vi "Disconnect.vi"(8 "error in (no error)":errorcluster, 11 "Ref":T1) -> (0 "error out":errorcluster)   [LabVIEW 2019, in "Ghost Bus Host Automation API.lvlib"]
uses:
  Ghost Bus Host Automation API.lvlib
  <vilib>/NI/STM/NI STM.lvlib
  <vilib>/NI/STM/TCP/Get Connection Reference (TCP).vi
  <vilib>/NI/STM/SubVIs/MetaDataElement.ctl
  <vilib>/NI/STM/TCP/TCP Connection Info.ctl
  Types/API Variables.ctl
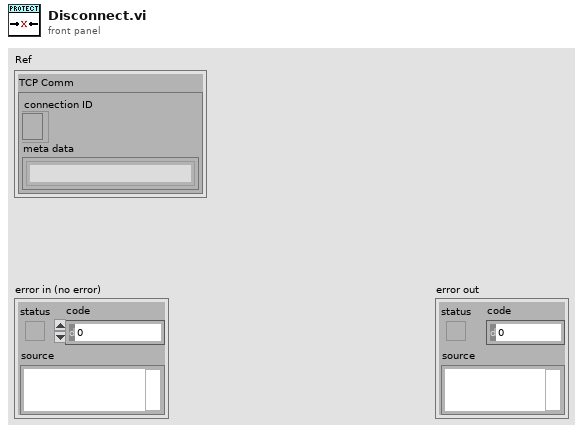
[diagram p1: front panel]
types:
  T1 = typedef "Ghost Bus Host Automation API.lvlib/API Variables.ctl" = cluster{"TCP Comm":T2}
  T2 = typedef "NI STM.lvlib/TCP Connection Info.ctl" = cluster{"connection ID":refnum<k5>, "meta data":T3[]}
  T3 = typedef "NI STM.lvlib/MetaDataElement.ctl" = string
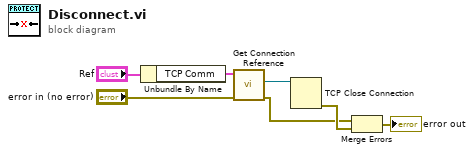
[diagram p0: block diagram]
diagram:
  n1 = Unbundle By Name("Ref") -> ("TCP Comm"=w1:T2)
  n2 = call-poly <vilib>:"Get Connection Reference.vi"("error in"="error in (no error)", "connection info in"=w1) -> ("error out"=w5:errorcluster, "connection ID out"=w7:refnum<k5>)  [unwired: 7 in, 1 out]
  n3 = TCP Close Connection(connection ID=w7) -> (error out=w6:errorcluster)  [unwired: 2 in, 1 out]
  n4 = Merge Errors(w5, w6) -> (→"error out":errorcluster)
